vi "GetType.vi"(8 "error in (no error)":errorcluster, 11 "Set Letter Time Msg":refnum<class "Set Letter Time Msg.lvclass">) -> (0 "error out":errorcluster, 2 "Data Sample":variant, 3 "Set Letter Time Msg":refnum<class "Set Letter Time Msg.lvclass">)   [LabVIEW 2015, in "CS++PPG.lvlib" / "Set Letter Time Msg.lvclass"]
uses:
  Set Letter Time Msg.lvclass
  Set Letter Time Msg.lvclass/Set Letter Time Msg.ctl
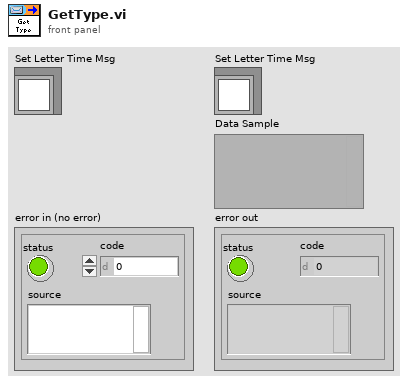
[diagram p1: front panel]
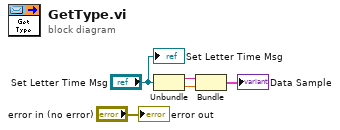
[diagram p0: block diagram]
diagram:
  n1 = Unbundle("Set Letter Time Msg") -> (w2:string, w1:dbl[unit])
  n2 = Bundle("Letter"=w2, "Time"=w1) -> (→"Data Sample":cluster{"Letter":string, "Time":dbl[unit]})  [unwired: 1 in]
  "error out" <- "error in (no error)"
  "Set Letter Time Msg" <- "Set Letter Time Msg"
